vi "Make JSON Object.vi"(6 "Pretty Print?":bool, 8 "error in (no error)":errorcluster, 9 "JSON Items":string[](array[string]), 11 "Item Names":string[](array[string])) -> (0 "error out":errorcluster, 3 "<JSON>":string caption="<JSON>Object")   [LabVIEW 2021, in "json.facade.lvlib"]
doc: "Format a JSON Object from named JSON elements."
uses:
  json.facade.lvlib
  jsontext/JSONtext.lvlib
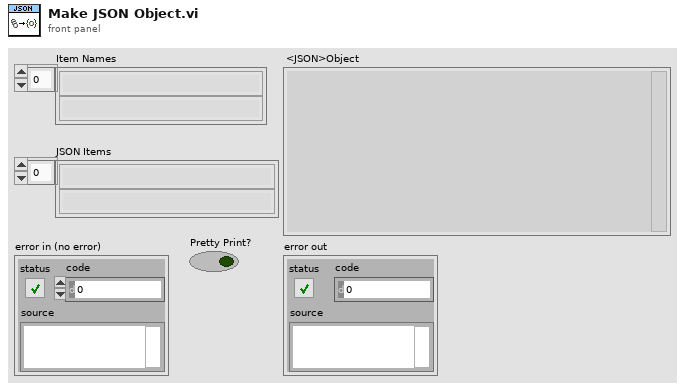
[diagram p1: front panel]
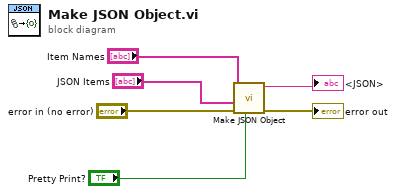
[diagram p0: block diagram]
diagram:
  n1 = call "Make JSON Object.vi"("Pretty Print?"="Pretty Print?", "error in (no error)"="error in (no error)", "JSON Items"="JSON Items", "Item Names"="Item Names") -> ("error out"=→"error out":errorcluster, "<JSON>"=→"<JSON>":string)  [unwired: 6 in]
